vi "take step.vi"(5 "approach?":bool=TRUE, 6 "motion":T1=enum."fast", 7 "blocking?":bool=TRUE, 8 "error in":errorcluster, 11 "actuator in":T2={"Actuator COM"="COM14", "Actuator type"=enum."Scientifica"}) -> (0 "error out":errorcluster, 3 "actuator out":T2={"Actuator COM"="COM14", "Actuator type"=enum."Scientifica"})   [LabVIEW 2015]
uses:
  pipette cleaning/pressure box/cleaning_soft/controls/scientifica_commands.ctl
  controls/scope_motion.ctl
  pipette cleaning/pressure box/cleaning_soft/controls/actuator_type.ctl
  pipette cleaning/pressure box/cleaning_soft/controls/actuator_cluster.ctl
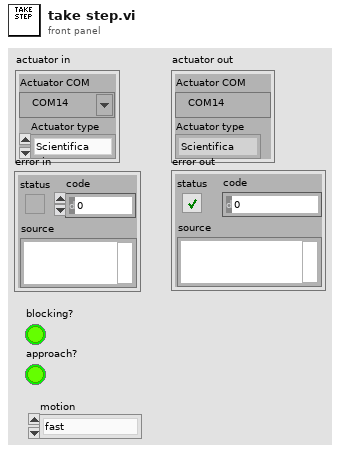
[diagram p1: front panel]
types:
  T1 = typedef "scope_motion.ctl" = enum16{"superSlow", "fast", "slow", "find slice speed", "slow_dualPatch"}
  T2 = typedef "actuator_cluster.ctl" = cluster{"Actuator COM":refnum<visa-resource-name>, "Actuator type":T3}
  T3 = typedef "actuator_type.ctl" = enum16{"Scientifica", "Sutter", "Demo", "Off"}
  T4 = typedef "scientifica_commands.ctl" = enum16{"ANGLE", "INSET", "FIRST", "ZERO", "Pz", "P", "absz", "ACC", "TOP", "STOP", "rel", "relz", "abs", "IN", "vj", "APROACH", "OBJS", "OBJU", "OUT", "OBJ", "OBJL", "SET", "OBJD", "STEP", "SETSTEP", "S", "UUX", "UUY", "UUZ"}
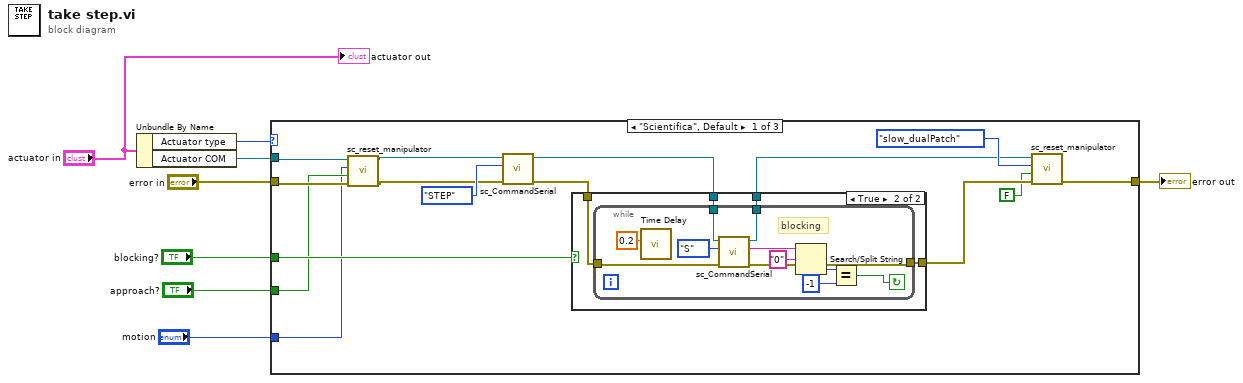
[diagram p0: block diagram]
diagram:
  n1 = Unbundle By Name("actuator in") -> ("Actuator type"=w7:T3, "Actuator COM"=w6:refnum<visa-resource-name>)
  n2 = case shown="\"Scientifica\", Default" w7 {
    tunnel: w6 -> [w19 _ _]
    tunnel: "error in" -> [w18 w41 w42]
    tunnel: [w16 w41 w42] -> w4
    tunnel: "blocking?" -> [w22 _ _]
    tunnel: "approach?" -> [w17 _ _]
    tunnel: "motion" -> [w13 _ _]
    frame "Scientifica", Default {
      n3 = call "sc_reset_manipulator.vi"("error in (no error)"=w18, "approach? (T = on)"=w17, "motion"=w13, "visa in"=w19) -> ("error out"=w14:errorcluster, "visa out"=w15:refnum<visa-resource-name>)  [unwired: 6 in]
      n4 = call "sc_CommandSerial.vi"("error in (no error)"=w14, "Scientifica commands"=scientifica_commands."STEP", "VISA handle"=w15) -> ("error out"=w21:errorcluster, "Dup. VISA handle"=w20:refnum<visa-resource-name>)  [unwired: 5 in, 2 out]
      n5 = case shown="True" w22 {
        tunnel: w21 -> [w25 w29]
        tunnel: [w25 w28] -> w10
        tunnel: w20 -> [w24 w27]
        tunnel: [w24 w26] -> w11
        frame False {
        }
        frame True {
          n6 = while {
            tunnel: w29 -> [w39]
            tunnel: [w33] -> w28
            tunnel: w27 -> [w31]
            tunnel: [w30] -> w26
            stop <- w34 continue-if-true
            # "blocking"
            n7 = call "Time Delay"("Delay Time (s)"=0.2) -> ()  [unwired: 10 in, 1 out]
            n8 = call "sc_CommandSerial.vi"("error in (no error)"=w39, "Scientifica commands"=scientifica_commands."S", "VISA handle"=w31) -> ("error out"=w33:errorcluster, "Response"=w37:string, "Dup. VISA handle"=w30:refnum<visa-resource-name>)  [unwired: 5 in, 1 out]
            n9 = Search/Split String(string=w37, search string/char (-)="0") -> (offset of match=w36:i32)  [unwired: 1 in, 2 out]
            n10 = Equal?(x=w36, y=-1) -> (x = y?=w34:bool)
          }
        }
      }
      n11 = call "sc_reset_manipulator.vi"("error in (no error)"=w10, "approach? (T = on)"=FALSE, "motion"=scope_motion."slow_dualPatch", "visa in"=w11) -> ("error out"=w16:errorcluster)  [unwired: 6 in, 1 out]
    }
    frame "Sutter" {
    }
    frame "Demo" {
    }
  }
  "error out" <- w4
  "actuator out" <- "actuator in"
